vi "Change Camera.vi"(8 "error in (no error)":errorcluster, 10 "New Camera":string, 11 "HIJ IMAQdx Camera Viewer In":refnum<class "HIJ Vision App IMAQdx Display.lvclass">) -> (0 "error out":errorcluster, 3 "HIJ IMAQdx Camera Viewer Out":refnum<class "HIJ Vision App IMAQdx Display.lvclass">)   [LabVIEW 2014, in "HIJ Vision App IMAQdx Display.lvlib" / "HIJ Vision App IMAQdx Display.lvclass"]
uses:
  HIJ Vision App IMAQdx Display.lvclass
  HIJ Vision Camera App/HIJ Vision Camera App/HIJ Vision Camera App.lvclass/HIJ Vision Camera App.ctl
  HIJ Vision Camera App Dialog/HIJ Vision Camera App Dialog Messages/New Camera Selection Msg/New Camera Selection Msg.lvclass/New Camera Selection Msg.ctl
  <vilib>/ActorFramework/Message Enqueuer/Message Enqueuer.lvclass/Message Enqueuer.ctl
  HIJ Vision Camera App/HIJ Vision Camera App/Read Dialog Enq.vi
  <vilib>/ActorFramework/Message Enqueuer/Enqueue.vi
  <vilib>/ActorFramework/Message Priority Queue/Priority Enqueue.vi
  HIJ Vision Camera App/HIJ Vision Camera App/HIJ Vision Camera App.lvclass
  <vilib>/ActorFramework/Message Enqueuer/Message Enqueuer.lvclass
  HIJ Vision Camera App Dialog/HIJ Vision Camera App Dialog Messages/New Camera Selection Msg/New Camera Selection Msg.lvclass
  Shared Code/Viewable Actor/ViewableActor/ViewableActor.lvclass
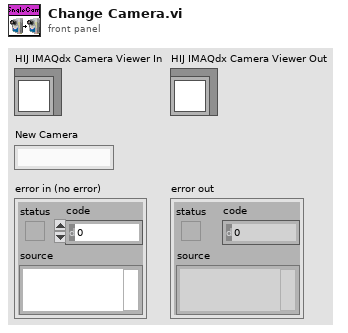
[diagram p1: front panel]
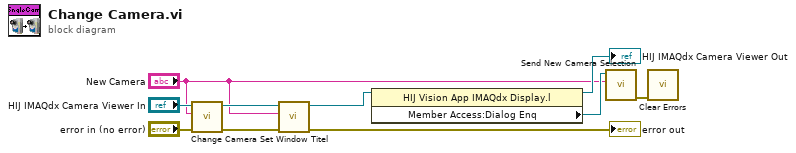
[diagram p0: block diagram]
diagram:
  n1 = call-parent "Change Camera.vi"("error in (no error)"="error in (no error)", "New Camera"="New Camera", "HIJ Vision Camera App In"="HIJ IMAQdx Camera Viewer In") -> ("error out"=w5:errorcluster, "HIJ Vision Camera App Out"=w6:refnum<class "HIJ Vision App IMAQdx Display.lvclass">)  [unwired: 7 in]
  n2 = call "Set Window Titel.vi"("error in (no error)"=w5, "Title"="New Camera", "ViewableActor in"=w6) -> ("error out"=→"error out":errorcluster, "ViewableActor out"=w8:refnum<class "HIJ Vision App IMAQdx Display.lvclass">)  [unwired: 7 in]
  n3 = property class="HIJ Vision App IMAQdx Display.l"(reference=w8) -> (reference out=→"HIJ IMAQdx Camera Viewer Out":refnum<class "HIJ Vision App IMAQdx Display.lvclass">, "Member Access:Dialog Enq"=w3:refnum<class "Message Enqueuer.lvclass">)  [unwired: 1 in, 1 out]
  n4 = call "Send New Camera Selection.vi"("New Camera Selection"="New Camera", "Message Enqueuer"=w3) -> ("error out"=w1:errorcluster)  [unwired: 8 in, 1 out]
  n5 = call <vilib>:"Clear Errors.vi"("error in (no error)"=w1) -> ()  [unwired: 5 in, 2 out]
